vi "get_visa_write_node_term.vi"(0 "Terms[] In":refnum<vi>[](array[refnum]), 11 "error in (no error)":errorcluster) -> (4 "Terms[]  Out":refnum<vi>[](array[refnum]), 6 "VISA In  Term":refnum<vi>, 8 "Error In Term":refnum<vi>, 10 "Error Out Term":refnum<vi>, 14 "Visa Out Term":refnum<vi>, 15 "error out":errorcluster)   [LabVIEW 2018]
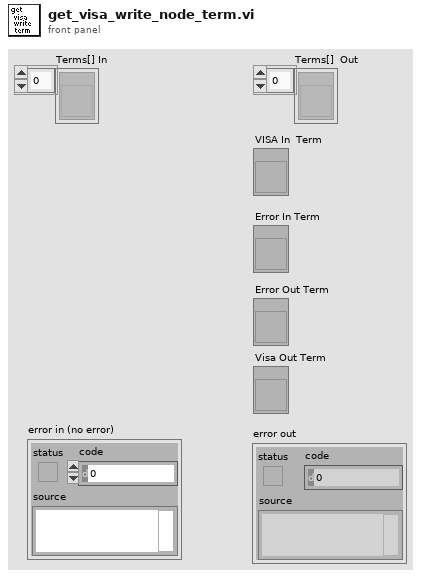
[diagram p1: front panel]
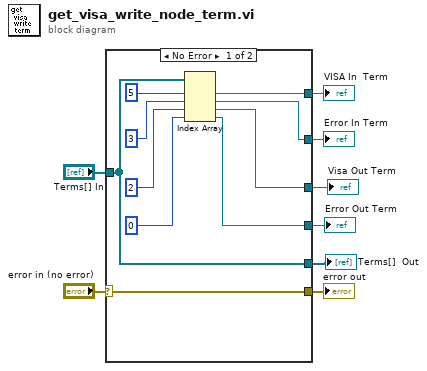
[diagram p0: block diagram]
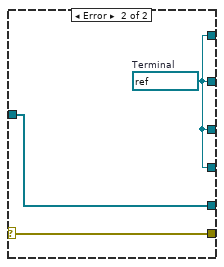
[diagram p2: hidden frame]
diagram:
  n1 = case shown="No Error" "error in (no error)" {
    selector: "error in (no error)" -> [w16 w21]
    tunnel: [w17 w19] -> w8
    tunnel: "Terms[] In" -> [w15 w20]
    tunnel: [w11 w19] -> w6
    tunnel: [w16 w21] -> w4
    tunnel: [w15 w20] -> w3
    tunnel: [w9 w19] -> w2
    tunnel: [w10 w19] -> w1
    frame No Error {
      n2 = Index Array(array=w15, index #1=5 ("index"), index #2=3 ("index"), index #3=2 ("index"), index #4=0 ("index")) -> (element #1=w17:refnum<vi>, element #2=w11:refnum<vi>, element #3=w10:refnum<vi>, element #4=w9:refnum<vi>)
    }
    frame Error {
      w19 = refnum<vi> refnum  # Terminal
    }
  }
  "VISA In  Term" <- w8
  "Error In Term" <- w6
  "error out" <- w4
  "Terms[]  Out" <- w3
  "Error Out Term" <- w2
  "Visa Out Term" <- w1
